vi "Error_Estimate.vi"(3 "Block No":i32=1, 4 "Sampling Frequency (Hz)":dbl, 5 "Data In":dbl[][](array[numeric])) -> (0 "Integral to 25%":dbl[](array[numeric]), 1 "Variance":dbl[](array[numeric]), 2 "Error Estimates":dbl[](array[numeric]))   [LabVIEW 2010]
uses:
  Globals/Meas_global.vi
panel:
  out "Mean":dbl[](array[numeric])
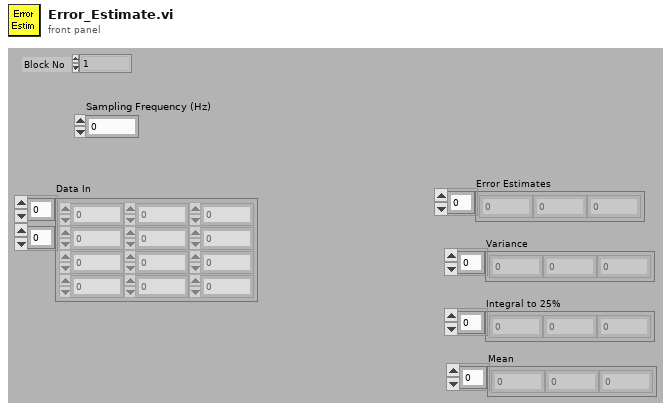
[diagram p1: front panel]
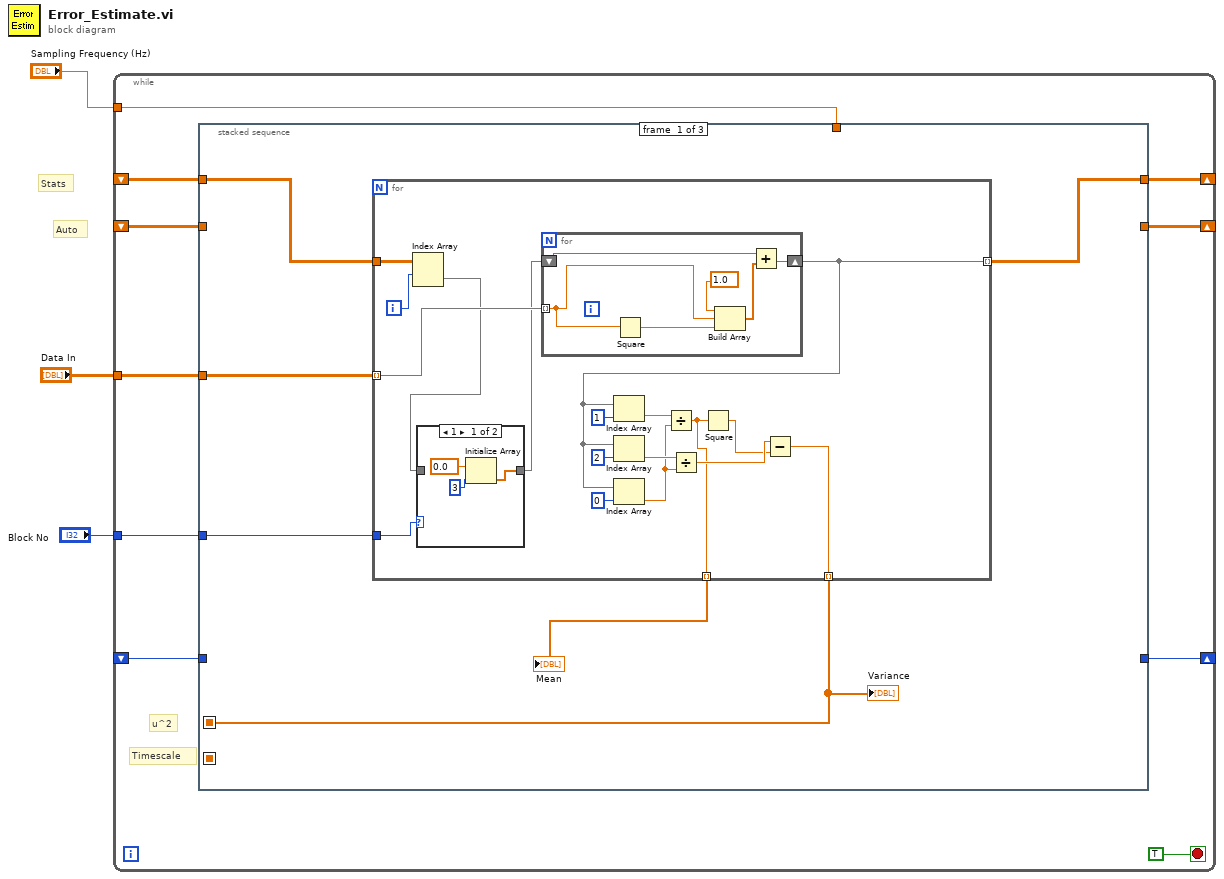
[diagram p0: block diagram]
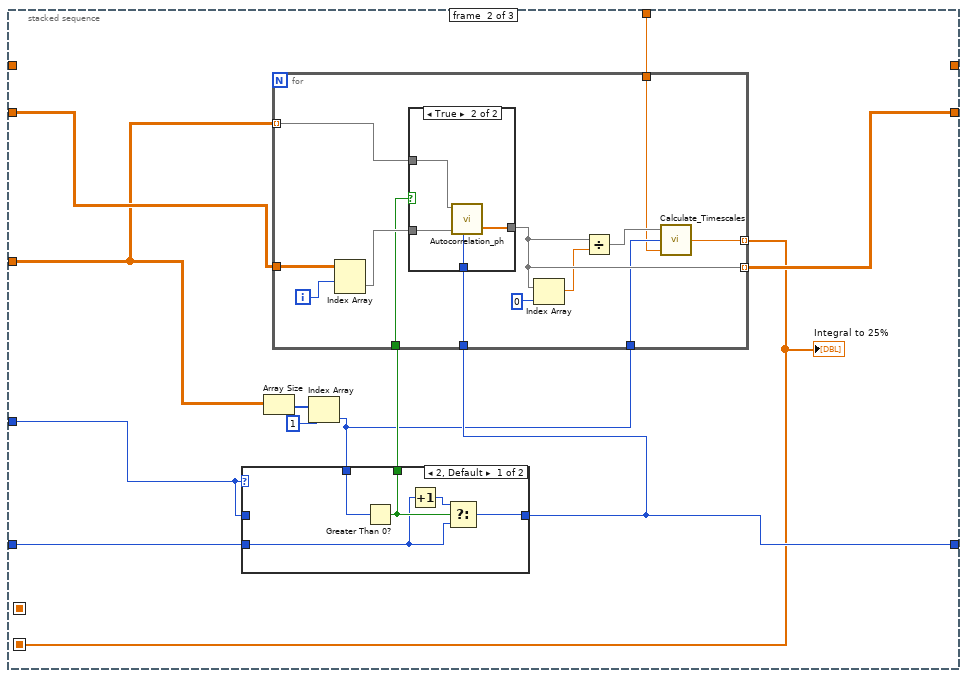
[diagram p3: hidden frame]
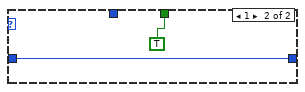
[diagram p4: hidden frame]
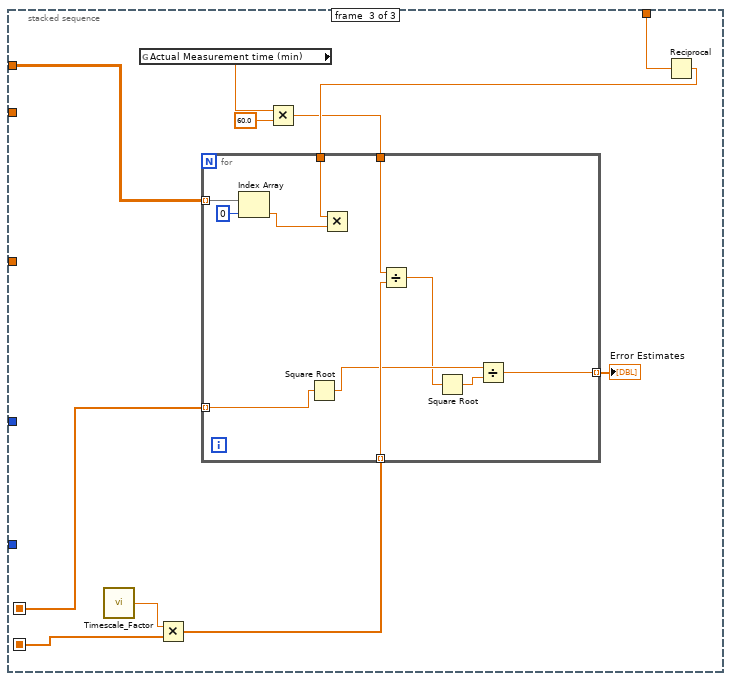
[diagram p6: hidden frame]
diagram:
  # "Auto"
  # "Stats"
  n1 = while {
    shift-right: [w11] -> _
    shift-left: _ -> [w12]
    tunnel: "Data In" -> [w13]
    tunnel: "Block No" -> [w10]
    shift-right: [w8] -> _
    shift-left: _ -> [w9]
    shift-right: [w6] -> _
    shift-left: _ -> [w7]
    tunnel: "Sampling Frequency (Hz)" -> [w4]
    stop <- TRUE stop-if-true
    # "Timescale"
    # "u^2"
    n2 = stacked-sequence {
      seq-local: [w15 _ _] -> [_ _ w88]
      seq-local: [_ w47 _] -> [_ _ w90]
      tunnel: w13 -> [w19 w50 _]
      tunnel: w12 -> [w17 _ w94]
      tunnel: [w18 _ _] -> w11
      tunnel: w10 -> [w16 w56 _]
      tunnel: w9 -> [_ w58 _]
      tunnel: [_ w57 _] -> w8
      tunnel: w7 -> [_ w55 _]
      tunnel: [_ w54 _] -> w6
      tunnel: w4 -> [_ w48 w93]
      frame #0 {
        n3 = for {
          tunnel: w19 -> [w36] mode=indexing
          tunnel: [w27] -> w18 mode=indexing
          tunnel: w17 -> [w34]
          tunnel: w16 -> [w31]
          tunnel: [w21] -> w15 mode=indexing
          tunnel: [w20] -> w14 mode=indexing
          i -> [w35]
          n4 = Index Array(array=w34, index (row)=w35) -> (element=w33:dbl[])  [unwired: 1 in]
          n5 = case shown="1" w31 {
            tunnel: [w37 w40] -> w32
            tunnel: w33 -> [_ w40]
            frame 1 {
              n6 = Initialize Array(0.0 ("Element Data"), 3 ("Dimension Size")) -> (w37:dbl[])
            }
            frame 2, Default {
            }
          }
          n7 = for {
            shift-right: [w45] -> w27
            shift-left: w32 -> [w46]
            tunnel: w36 -> [w42] mode=indexing
            n8 = Square(x=w42) -> (x^2=w41:dbl)
            n9 = Build Array(1.0 ("Input Element"), w42, w41) -> (w44:dbl[])
            n10 = Add(x=w46, y=w44) -> (x+y=w45:dbl[])
          }
          n11 = Index Array(array=w27, index=1) -> (element=w26:dbl)
          n12 = Index Array(array=w27, index=2) -> (element=w25:dbl)
          n13 = Index Array(array=w27, index=0) -> (element=w24:dbl)
          n14 = Divide(x=w26, y=w24) -> (x/y=w20:dbl)
          n15 = Divide(x=w25, y=w24) -> (x/y=w23:dbl)
          n16 = Square(x=w20) -> (x^2=w22:dbl)
          n17 = Subtract(x=w23, y=w22) -> (x-y=w21:dbl)
        }
        "Variance" <- w15
        "Mean" <- w14
      }
      frame #1 {
        n18 = Array Size(array=w50) -> (size(s)=w51:i32[])
        n19 = Index Array(array=w51, index=1) -> (element=w49:i32)
        n20 = case shown="2, Default" w56 {
          tunnel: [w60 w65] -> w54
          tunnel: w56 -> [_ w65]
          tunnel: [w63 TRUE] -> w53
          tunnel: w55 -> [w61 _]
          tunnel: w49 -> [w59 _]
          frame 2, Default {
            n21 = Greater Than 0?(x=w59) -> (x > 0?=w63:bool)
            n22 = Increment(x=w61) -> (x+1=w62:i32)
            n23 = Select(t=w62, s=w63, f=w61) -> (s? t:f=w60:i32)
          }
          frame 1 {
          }
        }
        n24 = for {
          tunnel: [w74] -> w57 mode=indexing
          tunnel: w58 -> [w76]
          tunnel: w53 -> [w72]
          tunnel: w54 -> [w71]
          tunnel: w50 -> [w70] mode=indexing
          tunnel: w49 -> [w68]
          tunnel: [w67] -> w47 mode=indexing
          tunnel: w48 -> [w66]
          i -> [w78]
          n25 = Index Array(array=w76, index (row)=w78) -> (element=w77:dbl[])  [unwired: 1 in]
          n26 = case shown="True" w72 {
            tunnel: w70 -> [_ w83]
            tunnel: w77 -> [w79 w82]
            tunnel: [w79 w81] -> w74
            tunnel: w71 -> [_ w80]
            frame False {
            }
            frame True {
              n27 = call "Autocorrelation_ph.vi"("X"=w83, "Autocorrelation of X"=w82, "Block No"=w80) -> ("Autocorrelation of X"=w81:dbl[])  [unwired: 2 in, 1 out]
            }
          }
          n28 = Index Array(array=w74, index=0 ("Index")) -> (element=w73:dbl)
          n29 = Divide(x=w74, y=w73) -> (x/y=w69:dbl[])
          n30 = call "Calculate_Timescales.vi"("Sampling Frequency (Hz)"=w66, "Autocorrelation length"=w68, "Autocorrelation"=w69) -> ("Time Scale estimate (s)"=w67:dbl)
        }
        "Integral to 25%" <- w47
      }
      frame #2 {
        n31 = call "Timescale_Factor.vi"() -> ("Factor to scale timescale by"=w91:dbl)
        n32 = global read "Meas_global.vi" "Actual Measurement time (min)"() -> (w86:dbl)
        n33 = Multiply(x=w91, y=w90) -> (x*y=w89:dbl[])
        n34 = Multiply(x=w86, y=60.0) -> (x*y=w84:dbl)
        n35 = Reciprocal(x=w93) -> (1/x=w92:dbl)
        n36 = for {
          tunnel: w94 -> [w105] mode=indexing
          tunnel: w92 -> [w103]
          tunnel: w89 -> [w101] mode=indexing
          tunnel: w88 -> [w100] mode=indexing
          tunnel: [w97] -> w87 mode=indexing
          tunnel: w84 -> [w95]
          n37 = Index Array(array=w105, index=0) -> (element=w102:dbl)
          n38 = Square Root(x=w100) -> (sqrt(x)=w99:dbl)
          n39 = Multiply(x=w103, y=w102) -> ()  [unwired: 1 out]
          n40 = Divide(x=w95, y=w101) -> (x/y=w98:dbl)
          n41 = Square Root(x=w98) -> (sqrt(x)=w96:dbl)
          n42 = Divide(x=w99, y=w96) -> (x/y=w97:dbl)
        }
        "Error Estimates" <- w87
      }
    }
  }
